vi "Set Initialization Data - gRPC Client.vi"(8 "error in":errorcluster, 11 "gRPC Client Tester in":refnum<class "gRPC Client Tester.lvclass">) -> (0 "error out":errorcluster, 3 "gRPC Client Tester out":refnum<class "gRPC Client Tester.lvclass">)   [LabVIEW 2019, in "gRPC Client Tester.lvclass"]
doc: "In this VI you can set the initialization data of a statically-linked subWorker."
uses:
  gRPC Client Tester.lvclass
  gRPC Client/gRPC Client/Initialization Data.ctl
  gRPC Client/gRPC Client/Response Cases.ctl
  <vilib>/addons/_Workers/Library/Case Label.ctl
  gRPC Client Tester.lvclass/gRPC Client Tester.ctl
  gRPC Client/gRPC Client/gRPC Client.lvclass
  C:/Program Files (x86)/National Instruments/LabVIEW 2019/vi.lib/addons/_Workers/Library/Classes/Worker/Worker.lvclass
  <vilib>/addons/_Workers/Library/Workers.lvlib
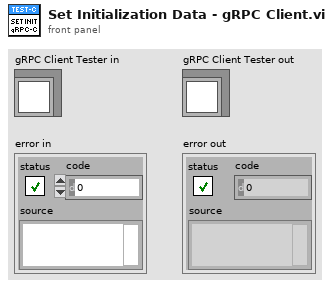
[diagram p1: front panel]
types:
  T1 = typedef "gRPC Client (template.proto).lvlib/gRPC Client.lvclass/Initialization Data.ctl" = cluster{"Response Cases":T2}
  T2 = typedef "gRPC Client (template.proto).lvlib/gRPC Client.lvclass/Response Cases.ctl" = cluster{"Connection Notify":T3, "Client Error":T3, "Msg_ToClient_1":T3, "Msg_ToClient_2":T3, "Msg_ToClient_3":T3, "Msg_ToClient_4":T3, "Msg_ToClient_5":T3, "Msg_ToClient_6":T3, "Msg_ToClient_7":T3, "Msg_ToClient_8":T3, "Msg_ToClient_9":T3}
  T3 = typedef "Workers.lvlib/Case Label.ctl" = string
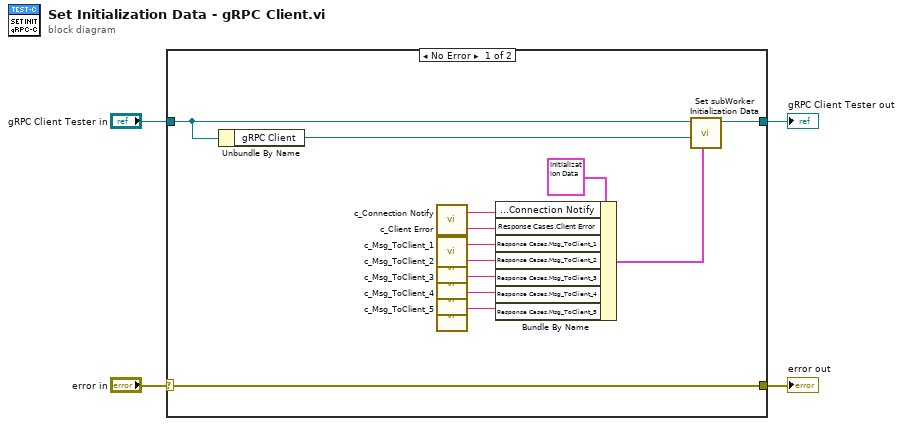
[diagram p0: block diagram]
diagram:
  n1 = case shown="No Error" "error in" {
    selector: "error in" -> [w17 w19]
    tunnel: [w17 w19] -> w3
    tunnel: [w15 w18] -> w2
    tunnel: "gRPC Client Tester in" -> [w14 w18]
    frame No Error {
      n2 = Unbundle By Name(w14) -> ("gRPC Client"=w16:refnum<class "gRPC Client.lvclass">)
      n3 = call "c_Connection Notify.vi"() -> ("Case Label"=w11:T3)  [unwired: 1 in]
      n4 = call "c_Client Error.vi"() -> ("Case Label"=w10:T3)  [unwired: 1 in]
      n5 = call "c_Msg_ToClient_1.vi"() -> ("Case Label"=w9:T3)  [unwired: 1 in]
      n6 = call "c_Msg_ToClient_2.vi"() -> ("Case Label"=w8:T3)  [unwired: 1 in]
      n7 = call "c_Msg_ToClient_3.vi"() -> ("Case Label"=w7:T3)  [unwired: 1 in]
      n8 = call "c_Msg_ToClient_4.vi"() -> ("Case Label"=w6:T3)  [unwired: 1 in]
      n9 = call "c_Msg_ToClient_5.vi"() -> ("Case Label"=w5:T3)  [unwired: 1 in]
      n10 = Bundle By Name(cluster=T1 {"Response Cases"={"Connection Notify"="", "Client Error"="", "Msg_ToClient_1"="", "Msg_ToClient_2"="", "Msg_ToClient_3"="", "Msg_ToClient_4"="", "Msg_ToClient_5"="", "Msg_ToClient_6"="", "Msg_ToClient_7"="", "Msg_ToClient_8"="", "Msg_ToClient_9"=""}} ("Initialization Data"), "Response Cases.Connection Notify"=w11, "Response Cases.Client Error"=w10, "Response Cases.Msg_ToClient_1"=w9, "Response Cases.Msg_ToClient_2"=w8, "Response Cases.Msg_ToClient_3"=w7, "Response Cases.Msg_ToClient_4"=w6, "Response Cases.Msg_ToClient_5"=w5) -> (w12:T1)
      n11 = call-dynamic "Set subWorker Initialization Data.vi"("Initialization Data"=w12, "subWorker"=w16, "Worker"=w14) -> ("Worker out"=w15:refnum<class "gRPC Client Tester.lvclass">)  [unwired: 8 in]
    }
    frame Error {
    }
  }
  "error out" <- w3
  "gRPC Client Tester out" <- w2
